vi "rate.vi"(4 "Scan Period":dbl format="%.2f", 5 "Previous Scan Value":dbl format="%.2f", 6 "Present scan array":dbl[](array[numeric]) format="%.2f", 7 "Value to Output":dbl format="%.2f", 8 "Ch Description":T2={"Ch Name"="Vib:NDE:MapCheck", "Type"="Run VI Named:", "Function"=enum."Analogue Input", "Ch State"=enum."On", "Calibration type"="Raw", "A"=0.15, "B"=10.0, "C"=0.0, "D"=0.0, "Comments"="MapCompare.vi", "Address"={"Main"=0, "Ch."=0, "Sub"=0, "Port Name"=""}, "String"="vibMapEastNDE.xls;VFD-E:Measured:RPM;VFD-E:Vibro:NDE(RMSmm/s)", "Duty"=65535} {"Duty" format="%016b"; "D" format="%#_5g"; "C" format="%#_5g"; "B" format="%#_5g"; "A" format="%#_5g"}, 9 "Ch names":string[](array[string])) -> (0 "Scan comment":string, 1 "Output":dbl format="%.3f", 3 "HelpText":string="Compares values retrieved from earlier channel with \"map\" of historic values, and warns if new values are out of spec.\nThis help text needs to be made dynamic.\nAcceptable radius (in Y axis units) is in A, minimum number of historic points is in B.")   [LabVIEW 2022 SP3]
uses:
  ADAM Client/Sub VIs/ADAM Controls/Ch_description_ADAM.ctl
  ADAM Client/Sub VIs/ADAM Controls/Module_type_ADAM.ctl
  ADAM Client/Sub VIs/ADAM Controls/Function_ADAM.ctl
  ADAM Client/Sub VIs/ADAM Controls/Channel_State.ctl
  ADAM Client/Sub VIs/ADAM Controls/Calib_type_ADAM.ctl
  ADAM Client/Sub VIs/ADAM Controls/Address.ctl
panel:
  in  "Ch State":T1
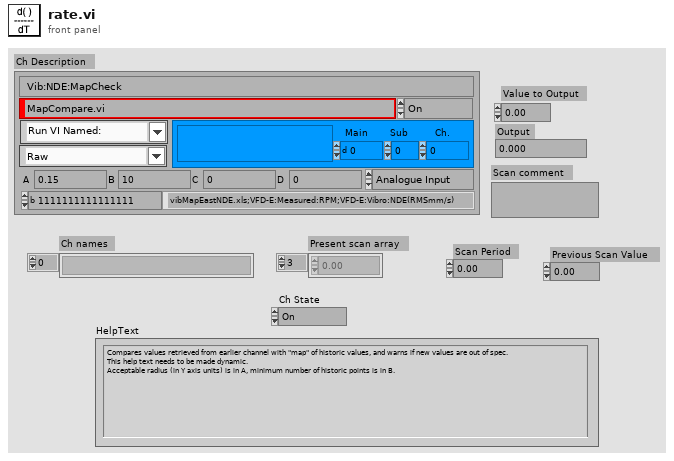
[diagram p1: front panel]
types:
  T1 = typedef "Channel_State.ctl" = enum16{"On", "Off", "Always On", "Always Off"}
  T2 = typedef "Ch_description_ADAM.ctl" = cluster{"Ch Name":string, "Type":T3, "Function":T4, "Ch State":T1, "Calibration type":T5, "A":dbl, "B":dbl, "C":dbl, "D":dbl, "Comments":string, "Address":T6, "String":string, "Duty":u16}
  T3 = typedef "Module_type_ADAM.ctl" = string
  T4 = typedef "Function_ADAM.ctl" = enum16{"Analogue Input", "Digital Input", "Event counter", "Event rate", "Analogue Output", "Digital Output", "Relay Output"}
  T5 = typedef "Calib_type_ADAM.ctl" = string
  T6 = typedef "Address.ctl" = cluster{"Main":i32, "Ch.":i32, "Sub":i32, "Port Name":string}
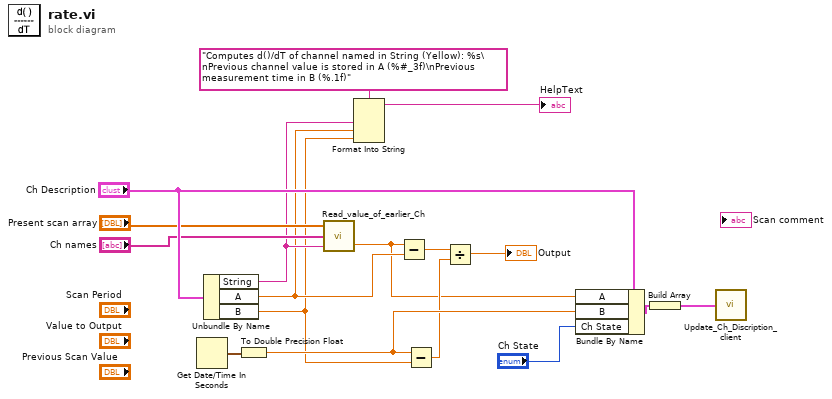
[diagram p0: block diagram]
diagram:
  n1 = Get Date/Time In Seconds() -> (seconds since 1Jan1904=w13:timestamp)
  n2 = Unbundle By Name("Ch Description") -> ("String"=w6:string, "A"=w4:dbl, "B"=w3:dbl)
  n3 = To Double Precision Float(number=w13) -> (double precision float=w12:dbl)
  n4 = call "Read_value_of_earlier_Ch.vi"("Desired Ch to Read"=w6, "Ch names"="Ch names", "Present scan array"="Present scan array") -> ("Value"=w2:dbl)  [unwired: 1 in, 1 out]
  n5 = Format Into String(format string="Computes d()/dT of channel named in String (Yellow): %s\nPrevious channel value is stored in A (%#_3f)\nPrevious measurement time in B (%.1f)" ("HelpText"), w6, w4, w3) -> (resulting string=→"HelpText":string)  [unwired: 2 in, 1 out]
  n6 = Subtract(x=w2, y=w4) -> (x-y=w11:dbl)
  n7 = Subtract(x=w12, y=w3) -> (x-y=w10:dbl)
  n8 = Divide(x=w11, y=w10) -> (x/y=→"Output":dbl)
  n9 = Bundle By Name(cluster="Ch Description", "A"=w2, "B"=w12, "Ch State"="Ch State") -> (w14:T2)
  n10 = Build Array(w14) -> (w15:T2[])
  n11 = call "Update_Ch_Discription_client.vi"("Channels to update In"=w15) -> ()  [unwired: 1 in]
